vi "Begin.vi"(8 "error in":errorcluster) -> (0 "error out":errorcluster)   [LabVIEW 2018]
doc: "Called before other user functions, this VI is expected to open initial I/O refnums, load in file data, and do all program initialization. Notice that the <B>error out</B> terminal is simply used for data flow. Wiring it to other structures or subVIs ensures that this VI runs first."
uses:
  <vilib>/Rock Robotics/WPI/DriverStation/WPI_DriverStationRobotMode2.ctl
  Robot Global Data.vi
  <vilib>/Rock Robotics/Network Tables/NT Write String Array.vi
  <vilib>/Rock Robotics/WPI/Utilities/WPI_GetSetVariantRefNum.vi
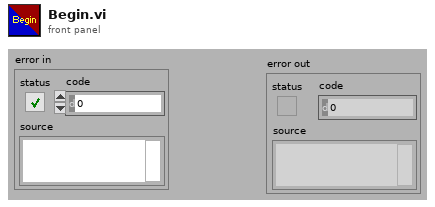
[diagram p1: front panel]
types:
  T1 = typedef "WPI_DriverStationRobotMode2.ctl" = enum16{"Autonomous Disabled", "Autonomous Enabled", "Teleop Disabled", "Teleop Enabled", "Disconnected", "Finish", "Test Disabled", "Test Enabled", "Emergency Stopped"}
  T2 = typedef "WPI_CompressorDevRef.ctl" = cluster{"DevStatus":errorcluster, "Pneumatics Control Module":u8}
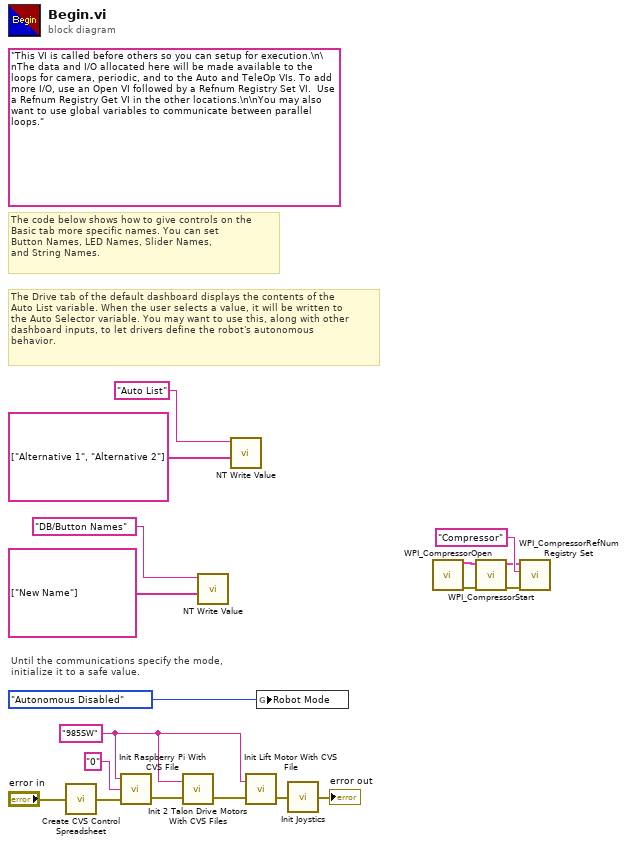
[diagram p0: block diagram]
diagram:
  w9 = "985SW" ("Robot ID")
  (unwired) "This VI is called before others so you can setup for execution.\n\nThe data and I/O allocated here will be made available to the loops for camera, periodic, and to the Auto and TeleOp VIs. To add more I/O, use an Open VI followed by a Refnum Registry Set VI.  Use a Refnum Registry Get VI in the other locations.\n\nYou may also want to use global variables to communicate between parallel loops."
  # "The Drive tab of the default dashboard displays the contents of the\nAuto List variable. When the user selects a value, it will be written to\nthe Auto Selector variable. You may want to use this, along with other\ndashboard inputs, to let drivers define the robot's autonomous\nbehavior."
  # "The code below shows how to give controls on the\nBasic tab more specific names. You can set\nButton Names, LED Names, Slider Names,\nand String Names."
  # "Until the communications specify the mode,\ninitialize it to a safe value."
  n1 = call "Create CVS Control Spreadsheet.vi"("error in"="error in") -> ("error out"=w11:errorcluster)
  n2 = call "Init Raspberry Pi With CVS File.vi"("error in"=w11, "Motor ID"="0", "Robot ID"=w9) -> ("error out"=w10:errorcluster)  [unwired: 1 out]
  n3 = call "Init 2 Talon Drive Motors With CVS Files.vi"("error in"=w10, "Robot ID"=w9) -> ("error out"=w8:errorcluster)  [unwired: 1 out]
  n4 = call-poly <vilib>:"NT Write Value.vi"("String Array"=string[] ["New Name"], "Name"="DB/Button Names") -> ()  [unwired: 9 in, 1 out]
  n5 = call-poly <vilib>:"NT Write Value.vi"("String Array"=string[] ["Alternative 1", "Alternative 2"], "Name"="Auto List") -> ()  [unwired: 9 in, 1 out]
  n6 = call "Init Lift Motor With CVS File.vi"("error in"=w8, "Robot ID"=w9) -> ("error out"=w7:errorcluster)  [unwired: 1 in]
  n7 = global write "Robot Global Data.vi" "Robot Mode"(WPI_DriverStationRobotMode2."Autonomous Disabled" ("Robot Mode")) -> ()
  n8 = call "Init Joystics.vi"("error in"=w7) -> ("error out"=→"error out":errorcluster)
  n9 = call <vilib>:"WPI_CompressorOpen.vi"() -> ("CompressorDevRef"=w5:T2, "error out"=w2:errorcluster)  [unwired: 14 in]
  n10 = call <vilib>:"WPI_CompressorStart.vi"("error in (no error)"=w2, "CompressorDevRef"=w5) -> ("error out"=w1:errorcluster, "CompressorDevRef"=w3:T2)  [unwired: 8 in]
  n11 = call <vilib>:"WPI_CompressorRefNum Registry Set.vi"("error in (no error)"=w1, "refnum name"="Compressor", "CompressorDevRef"=w3) -> ()  [unwired: 7 in, 2 out]
